vi "APC_9056_Signals.vi"() -> (0 "Starting Index":i32[](array[numeric]), 1 "9056_raster":string[](array[string]), 2 "signals per group":i32[](array[numeric]))   [LabVIEW 2020]
panel:
  # "NI9056"
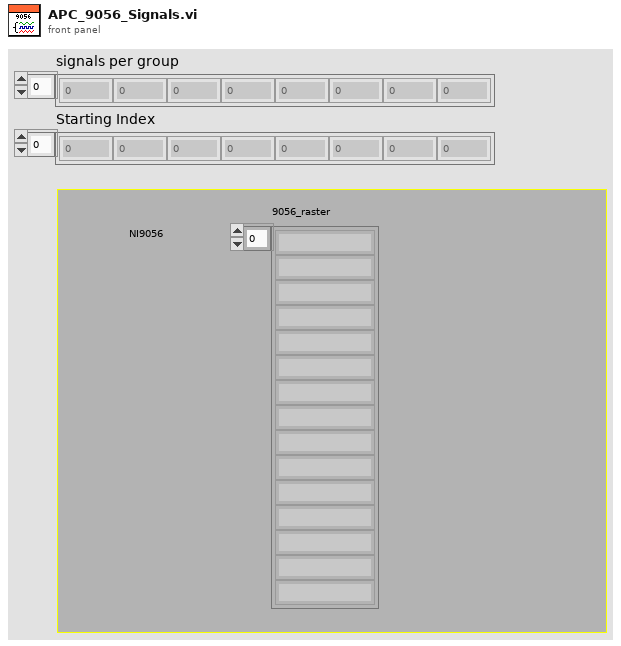
[diagram p1: front panel]
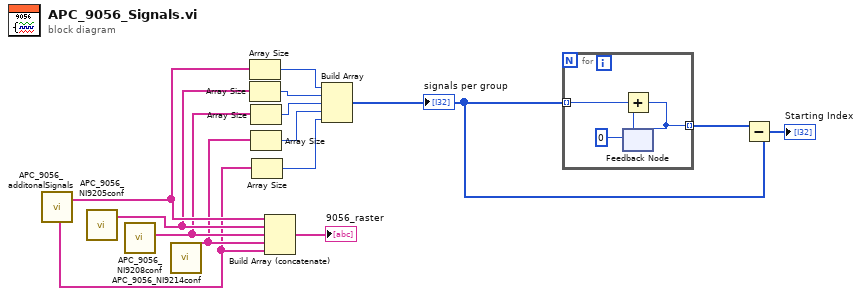
[diagram p0: block diagram]
diagram:
  n1 = call "APC_9056_additonalSignals.vi"() -> ("AdditionalTSSignalList_post"=w9:string[], "AdditionalTSSignalList_pre"=w13:string[])  [unwired: 2 in]
  n2 = call "APC_9056_NI9205conf.vi"() -> ("channels name out"=w12:string[])  [unwired: 5 out]
  n3 = call "APC_9056_NI9208conf.vi"() -> ("channels name out"=w11:string[])  [unwired: 5 out]
  n4 = call "APC_9056_NI9214conf.vi"() -> ("channels name out"=w10:string[])  [unwired: 5 in]
  n5 = Array Size(array=w13) -> (size(s)=w8:i32)
  n6 = Array Size(array=w12) -> (size(s)=w7:i32)
  n7 = Array Size(array=w11) -> (size(s)=w6:i32)
  n8 = Array Size(array=w10) -> (size(s)=w5:i32)
  n9 = Array Size(array=w9) -> (size(s)=w4:i32)
  n10 = Build Array (concatenate)(w13, w12, w11, w10, w9) -> (→"9056_raster":string[])
  n11 = Build Array(w8, w7, w6, w5, w4) -> (w1:i32[])
  "signals per group" <- w1
  n12 = for {
    tunnel: w1 -> [w18] mode=indexing
    tunnel: [w15] -> w3 mode=indexing
    n13 = feedback #1(0) -> (w17:i32)
    n14 = Add(x=w18, y=w17) -> (x+y=w15:i32)
    n15 = feedback-in #1(w15) -> ()
  }
  n16 = Subtract(x=w3, y=w1) -> (x-y=→"Starting Index":i32[])
